vi "[niSwitch] Close All.vi"() -> ()   [LabVIEW 2021]
panel:
  in  "Stop":bool
  in  "Close All session":bool
  out "Switch ref":refnum<k15>
  out "DropDownList[]":string[](array[string])
  # "NI Switch Sessions"
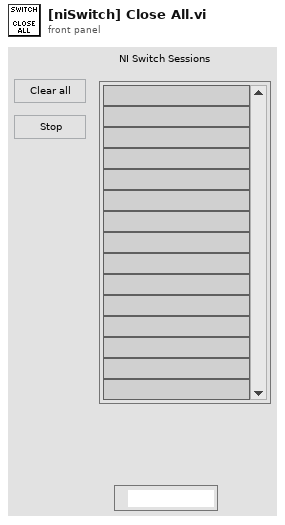
[diagram p1: front panel]
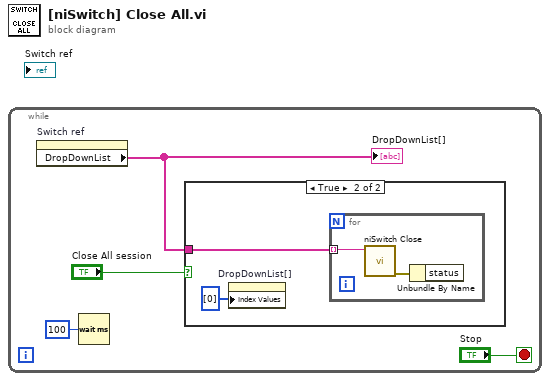
[diagram p0: block diagram]
diagram:
  n1 = while {
    stop <- "Stop" stop-if-true
    n2 = property on="Switch ref" class="IVIName"() -> ("DropDownList"=w2:string[])  [unwired: 2 in, 2 out]
    "DropDownList[]" <- w2
    n3 = Wait (ms)(milliseconds to wait=u32 100) -> ()  [unwired: 1 out]
    n4 = case shown="True" "Close All session" {
      tunnel: w2 -> [_ w6]
      frame False {
      }
      frame True {
        n5 = property on="DropDownList[]" class="Arr (strict)"("Index Values"=u32[] [0]) -> ()  [unwired: 2 in, 2 out]
        n6 = for {
          tunnel: w6 -> [w8] mode=indexing
          n7 = call <instrlib>:"niSwitch Close.vi"("instrument handle"=w8) -> ("error out"=w7:errorcluster)  [unwired: 10 in]
          n8 = Unbundle By Name(w7) -> ()  [unwired: 1 out]
        }
      }
    }
  }
